vi "Get_properties.vi"(8 "Keyword":string, 9 "Section":string, 11 "properties.ini":path) -> (0 "error":bool, 2 "number":dbl format="%.3g", 3 "string":string)   [LabVIEW 2011]
uses:
  <vilib>/Utility/config.llb/Read Key (String).vi
  <vilib>/Utility/config.llb/NI_LVConfig.lvlib
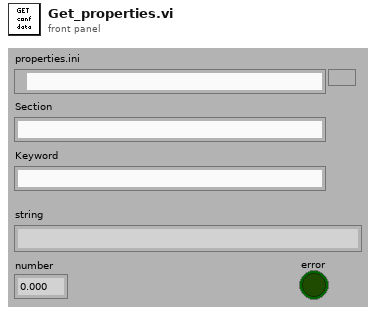
[diagram p1: front panel]
types:
  T1 = typedef "NI_LVConfig.lvlib/Config Data RefNum.ctl" = refnum<k1>
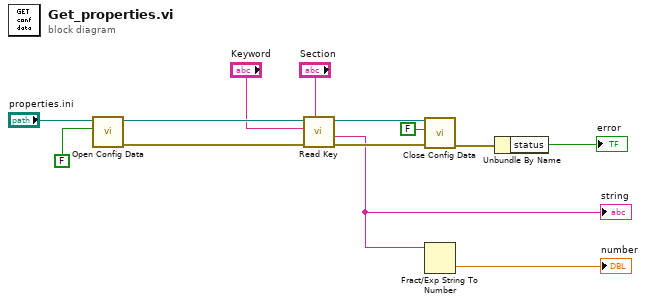
[diagram p0: block diagram]
diagram:
  n1 = call <vilib>:"Open Config Data.vi"("create file if necessary (T)"=FALSE, "configuration file path"="properties.ini") -> ("error out"=w10:errorcluster, "refnum"=w11:T1)  [unwired: 7 in, 1 out]
  n2 = call-poly <vilib>:"Read Key.vi"("section"="Section", "error in (no error)"=w10, "key"="Keyword", "refnum"=w11) -> ("error out"=w8:errorcluster, "value"=w3:string, "refnum out"=w9:T1)  [unwired: 4 in, 1 out]
  "string" <- w3
  n3 = call <vilib>:"Close Config Data.vi"("error in (no error)"=w8, "write file if changed (T)"=FALSE, "refnum"=w9) -> ("error out"=w7:errorcluster)  [unwired: 7 in, 1 out]
  n4 = Fract/Exp String To Number(string=w3) -> (number=→"number":dbl)  [unwired: 3 in, 1 out]
  n5 = Unbundle By Name(w7) -> ("status"=→"error":bool)
